vi "Zeiss File Header.vi"(0 "refnum":refnum<file>, 1 "Notes":string, 2 "Other detectors":T1, 5 "task":refnum<k21>, 7 "Resolution and scan":T5={"X resolution"=1, "Y resolution"=1, "AI oversampling"=1, "Read AI delay"=1, "Scan speed"=1, "Actual AO rate"=1.0, "Frame line rampdown ratio"=1.0, "X min (V)"=0.0, "X max (V)"=0.0}, 9 "AI channels":T4, 11 "error in":errorcluster, 12 "SEM parameters":T2={"Detector A"="", "Detector B"="Detecter B name", "Brightness A"=0.0, "Contrast A"=0.0, "Brightness B"=0.0, "Contrast B"=0.0, "Magnification"=0.0, "Pixel size"=0.0, "Working distance"=0.0, "EHT"=0.0, "Aperture"=0, "High current mode"=0, "Probe current"=0.0, "Scan rotation"=0.0, "Chamber vac"=0.0, "Gun vac"=0.0, "Beam shift X"=0.0, "Beam shift Y"=0.0, "Stig X"=0.0, "Stig Y"=0.0, "Alignment X"=0.0, "Alignment Y"=0.0, "Stage X"=0.0, "Stage Y"=0.0, "Stage Z"=0.0, "Stage T"=0.0, "Stage R"=0.0, "Stage M"=0.0}, 13 "FIB parameters":T3) -> (4 "dup refnum":refnum<file>, 6 "task out":refnum<k21>, 15 "error out":errorcluster)   [LabVIEW 2012]
uses:
  <resource>/objmgr/daqmx.rc
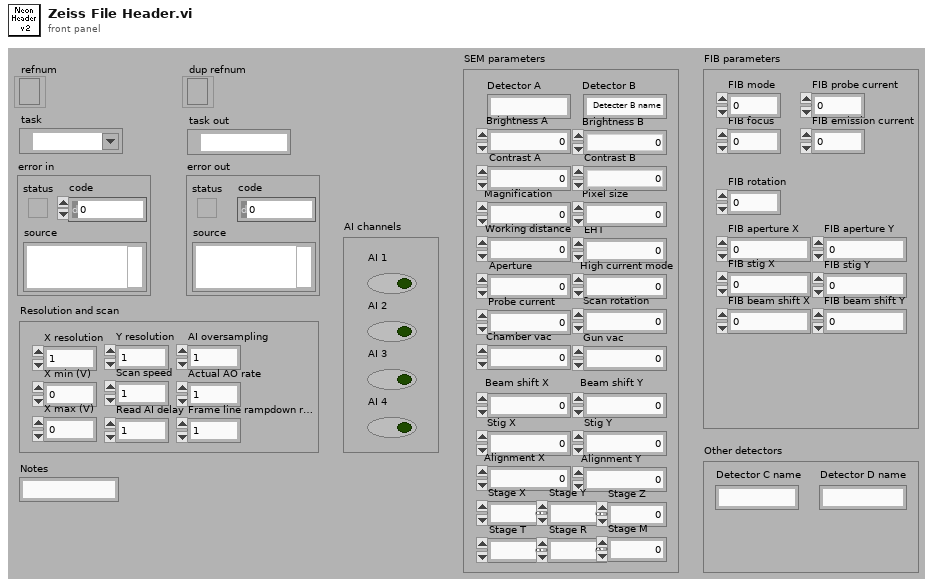
[diagram p1: front panel]
types:
  T1 = cluster{"Detector C name":string, "Detector D name":string}
  T2 = cluster{"Detector A":string, "Detector B":string, "Brightness A":sgl, "Contrast A":sgl, "Brightness B":sgl, "Contrast B":sgl, "Magnification":sgl, "Pixel size":sgl, "Working distance":sgl, "EHT":sgl, "Aperture":u8, "High current mode":u8, "Probe current":sgl, "Scan rotation":sgl, "Chamber vac":sgl, "Gun vac":sgl, "Beam shift X":sgl, "Beam shift Y":sgl, "Stig X":sgl, "Stig Y":sgl, "Alignment X":sgl, "Alignment Y":sgl, "Stage X":sgl, "Stage Y":sgl, "Stage Z":sgl, "Stage T":sgl, "Stage R":sgl, "Stage M":sgl}
  T3 = cluster{"FIB mode":u8, "FIB focus":sgl, "FIB probe current":u8, "FIB emission current":sgl, "FIB rotation":sgl, "FIB aperture X":sgl, "FIB aperture Y":sgl, "FIB stig X":sgl, "FIB stig Y":sgl, "FIB beam shift X":sgl, "FIB beam shift Y":sgl}
  T4 = cluster{"AI 1":bool, "AI 2":bool, "AI 3":bool, "AI 4":bool}
  T5 = cluster{"X resolution":u32, "Y resolution":u32, "AI oversampling":u16, "Read AI delay":i16, "Scan speed":u8, "Actual AO rate":dbl, "Frame line rampdown ratio":dbl, "X min (V)":dbl, "X max (V)":dbl}
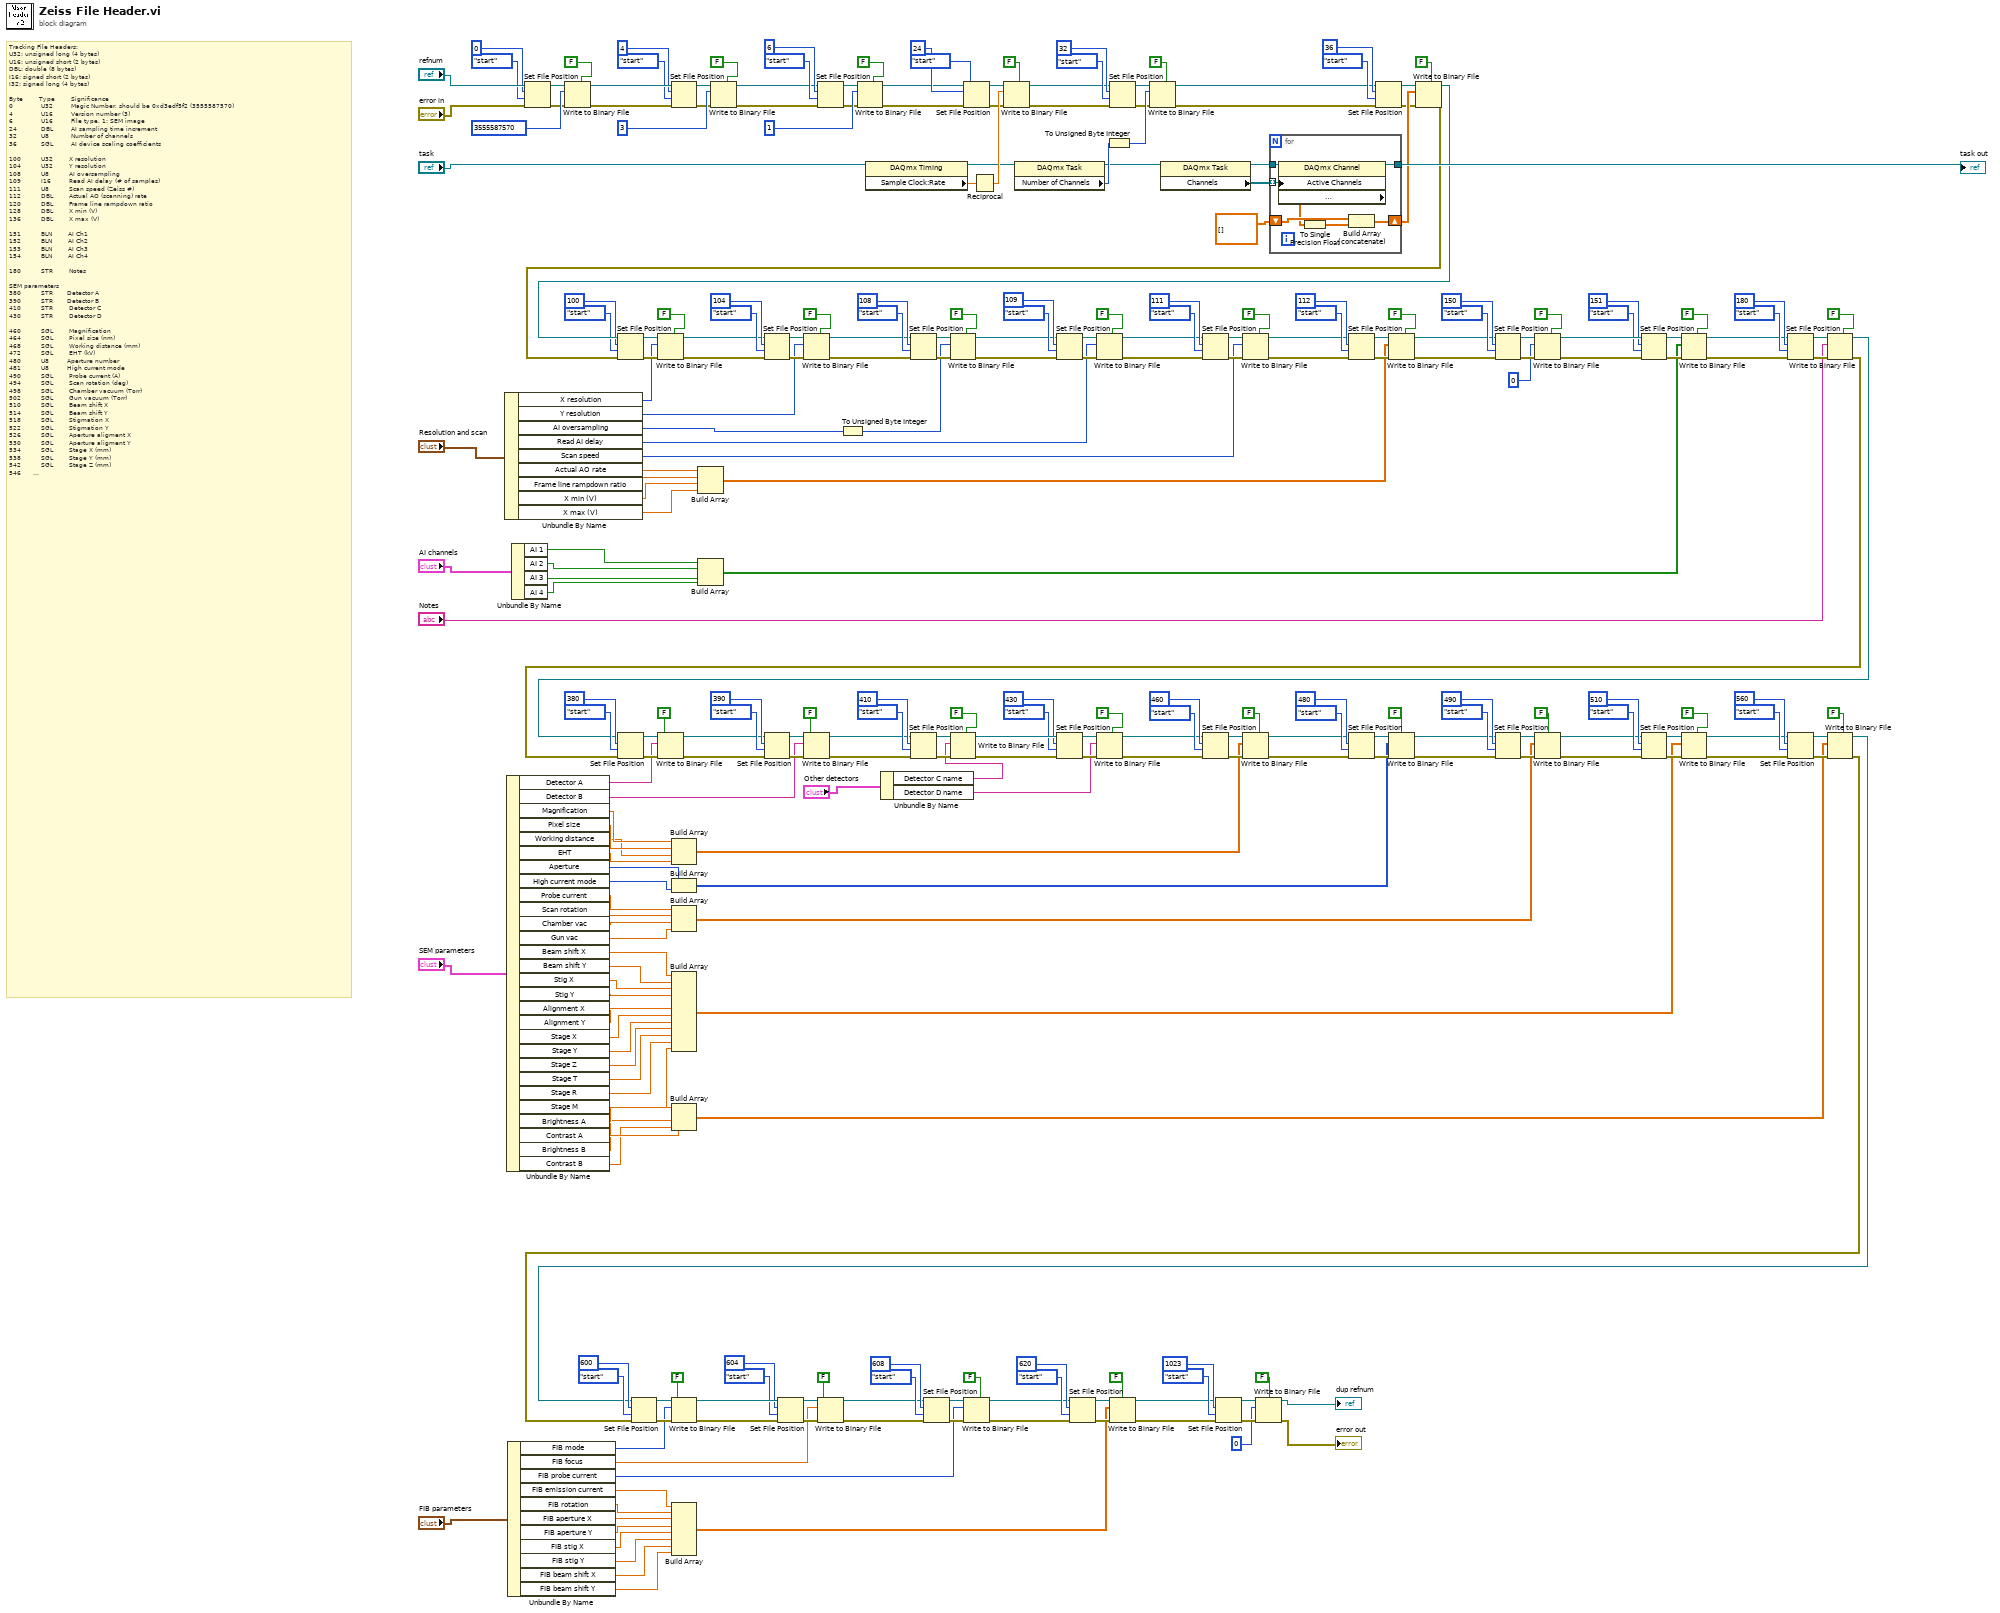
[diagram p0: block diagram]
diagram:
  # "Tracking File Headers:\nU32: unsigned long (4 bytes)\nU16: unsigned short (2 bytes)\nDBL: double (8 bytes)\nI16: signed short (2 bytes)\nI32: signed long (4 bytes)\n\nByte\t       Type\t\t      Significance\n0              U32\t        Magic Number, should be 0xd3edf5f2 (3555587570)\n4   \t          U16\t        Version number (3)\n6   \t          U16\t        File type. 1: SEM image\n24     \t      DBL         AI sampling time increment\n32     \t      U8           Number of channels\n36            SGL         AI device scaling coefficients\n\n100          U32        X resolution\n104          U32        Y resolution\n108          U8          AI oversampling\n109          I16         Read AI delay (# of samples)\n111          U8          Scan speed (Zeiss #)\n112          DBL        Actual AO (scanning) rate\n120          DBL        Frame line rampdown ratio\n128          DBL        X min (V)\n136          DBL        X max (V)\n\n151          BLN        AI Ch1          \n152          BLN        AI Ch2\n153          BLN        AI Ch3\n154          BLN        AI Ch4\n \n180          STR        Notes\n\nSEM parameters\n380          STR       Detector A\n390          STR       Detector B\n410          STR        Detector C\n430          STR        Detector D\n\n460          SGL        Magnification\n464          SGL        Pixel size (nm)\n468          SGL        Working distance (mm)\n472          SGL        EHT (kV)\n480          U8         Aperture number\n481          U8         High current mode\n490          SGL        Probe current (A)\n494          SGL        Scan rotation (deg)\n498          SGL        Chamber vacuum (Torr)\n502          SGL        Gun vacuum (Torr)\n510          SGL        Beam shift X\n514          SGL        Beam shift Y\n518          SGL        Stigmation X\n522          SGL        Stigmation Y\n526          SGL        Aperture aligment X\n530          SGL        Aperture aligment Y\n534          SGL        Stage X (mm)\n538          SGL        Stage Y (mm)\n542          SGL        Stage Z (mm)\n546          SGL        Stage T (deg)\n550          SGL        Stage R (deg)\n554          SGL        Stage M (mm)\n560          SGL        Brightness (%), detector A\n564          SGL        Contrast (%),  detector A\n568          SGL        Brightness (%), detector B\n572          SGL        Contrast (%),  detector B\n\n\nFIB parameters\n600          U8         Mode\n604          SGL        Focus (V)\n608          U8         Probe current number\n620          SGL        Emission current (A)\n624          SGL        rotation (deg)\n628          SGL        Aperture alignment X\n632          SGL        Aperture alignment Y\n636          SGL        Stigmation X\n640          SGL        Stigmation Y\n644          SGL        Beam shift X (um)\n648          SGL        Beam shift Y (um)\n\n\n1000        DBL         File length\n\n1024        I16          1-D array of n channels of unscaled measurement from DAQ"
  n1 = Unbundle By Name("Resolution and scan") -> ("X resolution"=w177:u32, "Y resolution"=w176:u32, "AI oversampling"=w175:u16, "Read AI delay"=w174:i16, "Scan speed"=w173:u8, "Actual AO rate"=w79:dbl, "Frame line rampdown ratio"=w78:dbl, "X min (V)"=w77:dbl, "X max (V)"=w76:dbl)
  n2 = Unbundle By Name("SEM parameters") -> ("Detector A"=w86:string, "Detector B"=w85:string, "Magnification"=w35:sgl, "Pixel size"=w34:sgl, "Working distance"=w33:sgl, "EHT"=w32:sgl, "Aperture"=w95:u8, "High current mode"=w94:u8, "Probe current"=w48:sgl, "Scan rotation"=w47:sgl, "Chamber vac"=w46:sgl, "Gun vac"=w45:sgl, "Beam shift X"=w71:sgl, "Beam shift Y"=w70:sgl, "Stig X"=w25:sgl, "Stig Y"=w24:sgl, "Alignment X"=w23:sgl, "Alignment Y"=w22:sgl, "Stage X"=w20:sgl, "Stage Y"=w19:sgl, "Stage Z"=w18:sgl, "Stage T"=w17:sgl, "Stage R"=w16:sgl, "Stage M"=w15:sgl, "Brightness A"=w84:sgl, "Contrast A"=w83:sgl, "Brightness B"=w81:sgl, "Contrast B"=w82:sgl)
  n3 = Unbundle By Name("FIB parameters") -> ("FIB mode"=w98:u8, "FIB focus"=w97:sgl, "FIB probe current"=w96:u8, "FIB emission current"=w12:sgl, "FIB rotation"=w11:sgl, "FIB aperture X"=w10:sgl, "FIB aperture Y"=w9:sgl, "FIB stig X"=w8:sgl, "FIB stig Y"=w7:sgl, "FIB beam shift X"=w6:sgl, "FIB beam shift Y"=w5:sgl)
  n4 = Unbundle By Name("AI channels") -> ("AI 1"=w40:bool, "AI 2"=w39:bool, "AI 3"=w38:bool, "AI 4"=w37:bool)
  n5 = Set File Position(offset (in bytes) (0)=0 ("pos offset (0)"), refnum="refnum", from (0:start)=enum16{"start", "end", "current"}."start" ("pos mode (0:2)"), error in="error in") -> (refnum out=w237:refnum<file>, error out=w236:errorcluster)
  n6 = Write to Binary File(file (use dialog)=w237, data=u32 3555587570, error in=w236, 5:FALSE ("prepend array or string size? (T)")) -> (refnum out=w289:refnum<file>, error out=w286:errorcluster)  [unwired: 3 out]
  n7 = Set File Position(offset (in bytes) (0)=4 ("pos offset (0)"), refnum=w289, from (0:start)=enum16{"start", "end", "current"}."start" ("pos mode (0:2)"), error in=w286) -> (refnum out=w240:refnum<file>, error out=w239:errorcluster)
  n8 = Build Array(w35, w34, w33, w32) -> (w31:sgl[])
  n9 = Build Array(w95, w94) -> (w28:u8[])
  n10 = Build Array(w48, w47, w46, w45) -> (w27:sgl[])
  n11 = Build Array(w71, w70, w25, w24, w23, w22, w20, w19, w18, w17, w16, w15) -> (w26:sgl[])
  n12 = Build Array(w84, w83, w81, w82) -> (w21:sgl[])
  n13 = Build Array(w12, w11, w10, w9, w8, w7, w6, w5) -> (w4:sgl[])
  n14 = Build Array(w79, w78, w77, w76) -> (w75:dbl[])
  n15 = Build Array(w40, w39, w38, w37) -> (w36:bool[])
  n16 = Write to Binary File(file (use dialog)=w240, data=u16 3, error in=w239, 5:FALSE ("prepend array or string size? (T)")) -> (refnum out=w280:refnum<file>, error out=w279:errorcluster)  [unwired: 3 out]
  n17 = Set File Position(offset (in bytes) (0)=6 ("pos offset (0)"), refnum=w280, from (0:start)=enum16{"start", "end", "current"}."start" ("pos mode (0:2)"), error in=w279) -> (refnum out=w243:refnum<file>, error out=w242:errorcluster)
  n18 = To Unsigned Byte Integer(number=w175) -> (unsigned 8bit integer=w72:u8)
  n19 = Write to Binary File(file (use dialog)=w243, data=u16 1, error in=w242, 5:FALSE ("prepend array or string size? (T)")) -> (refnum out=w275:refnum<file>, error out=w274:errorcluster)  [unwired: 3 out]
  n20 = property class="DAQmx Timing"(reference="task") -> (reference out=w271:refnum<k21>, "Sample Clock:Rate"=w273:dbl)  [unwired: 1 in, 1 out]
  n21 = Unbundle By Name("Other detectors") -> ("Detector C name"=w53:string, "Detector D name"=w52:string)
  n22 = Set File Position(offset (in bytes) (0)=24 ("pos offset (0)"), refnum=w275, from (0:start)=enum16{"start", "end", "current"}."start" ("pos mode (0:2)"), error in=w274) -> (refnum out=w246:refnum<file>, error out=w245:errorcluster)
  n23 = Reciprocal(x=w273) -> (1/x=w272:dbl)
  n24 = Write to Binary File(file (use dialog)=w246, data=w272, error in=w245, 5:FALSE ("prepend array or string size? (T)")) -> (refnum out=w268:refnum<file>, error out=w267:errorcluster)  [unwired: 3 out]
  n25 = property class="DAQmx Task"(reference=w271) -> (reference out=w265:refnum<k21>, "Number of Channels"=w266:u32)  [unwired: 1 in, 1 out]
  n26 = To Unsigned Byte Integer(number=w266) -> (unsigned 8bit integer=w258:u8)
  n27 = Set File Position(offset (in bytes) (0)=32 ("pos offset (0)"), refnum=w268, from (0:start)=enum16{"start", "end", "current"}."start" ("pos mode (0:2)"), error in=w267) -> (refnum out=w249:refnum<file>, error out=w248:errorcluster)
  n28 = Write to Binary File(file (use dialog)=w249, data=w258, error in=w248, 5:FALSE ("prepend array or string size? (T)")) -> (refnum out=w262:refnum<file>, error out=w261:errorcluster)  [unwired: 3 out]
  n29 = property class="DAQmx Task"(reference=w265) -> (reference out=w257:refnum<k21>, "Channels"=w255:refnum<k21>[])  [unwired: 1 in, 1 out]
  n30 = for {
    tunnel: [w298] -> w256
    tunnel: w257 -> [w297]
    tunnel: w255 -> [w296] mode=indexing
    shift-right: [w295] -> w254
    shift-left: sgl[][] [] -> [w294]
    n31 = property class="DAQmx Channel"(reference=w297, "Active Channels"=w296) -> (reference out=w298:refnum<k21>, "Analog Input:General Properties:Advanced:Device Scaling Coefficients:Device Scaling Coefficients"=w293:dbl[])  [unwired: 1 in, 1 out]
    n32 = To Single Precision Float(number=w293) -> (single precision float=w292:sgl[])
    n33 = Build Array (concatenate)(w294, w292) -> (w295:sgl[][])
  }
  "task out" <- w256
  n34 = Set File Position(offset (in bytes) (0)=36 ("pos offset (0)"), refnum=w262, from (0:start)=enum16{"start", "end", "current"}."start" ("pos mode (0:2)"), error in=w261) -> (refnum out=w252:refnum<file>, error out=w251:errorcluster)
  n35 = Write to Binary File(file (use dialog)=w252, data=w254, error in=w251, 5:FALSE ("prepend array or string size? (T)")) -> (refnum out=w234:refnum<file>, error out=w233:errorcluster)  [unwired: 3 out]
  n36 = Set File Position(offset (in bytes) (0)=100 ("pos offset (0)"), refnum=w234, from (0:start)=enum16{"start", "end", "current"}."start" ("pos mode (0:2)"), error in=w233) -> (refnum out=w226:refnum<file>, error out=w227:errorcluster)
  n37 = Write to Binary File(file (use dialog)=w226, data=w177, error in=w227, 5:FALSE ("prepend array or string size? (T)")) -> (refnum out=w203:refnum<file>, error out=w202:errorcluster)  [unwired: 3 out]
  n38 = Set File Position(offset (in bytes) (0)=104 ("pos offset (0)"), refnum=w203, from (0:start)=enum16{"start", "end", "current"}."start" ("pos mode (0:2)"), error in=w202) -> (refnum out=w219:refnum<file>, error out=w218:errorcluster)
  n39 = Write to Binary File(file (use dialog)=w219, data=w176, error in=w218, 5:FALSE ("prepend array or string size? (T)")) -> (refnum out=w205:refnum<file>, error out=w204:errorcluster)  [unwired: 3 out]
  n40 = Set File Position(offset (in bytes) (0)=108 ("pos offset (0)"), refnum=w205, from (0:start)=enum16{"start", "end", "current"}."start" ("pos mode (0:2)"), error in=w204) -> (refnum out=w216:refnum<file>, error out=w217:errorcluster)
  n41 = Write to Binary File(file (use dialog)=w216, data=w72, error in=w217, 5:FALSE ("prepend array or string size? (T)")) -> (refnum out=w207:refnum<file>, error out=w206:errorcluster)  [unwired: 3 out]
  n42 = Set File Position(offset (in bytes) (0)=109 ("pos offset (0)"), refnum=w207, from (0:start)=enum16{"start", "end", "current"}."start" ("pos mode (0:2)"), error in=w206) -> (refnum out=w209:refnum<file>, error out=w208:errorcluster)
  n43 = Write to Binary File(file (use dialog)=w209, data=w174, error in=w208, 5:FALSE ("prepend array or string size? (T)")) -> (refnum out=w196:refnum<file>, error out=w195:errorcluster)  [unwired: 3 out]
  n44 = Set File Position(offset (in bytes) (0)=111 ("pos offset (0)"), refnum=w196, from (0:start)=enum16{"start", "end", "current"}."start" ("pos mode (0:2)"), error in=w195) -> (refnum out=w198:refnum<file>, error out=w197:errorcluster)
  n45 = Write to Binary File(file (use dialog)=w198, data=w173, error in=w197, 5:FALSE ("prepend array or string size? (T)")) -> (refnum out=w189:refnum<file>, error out=w188:errorcluster)  [unwired: 3 out]
  n46 = Set File Position(offset (in bytes) (0)=112 ("pos offset (0)"), refnum=w189, from (0:start)=enum16{"start", "end", "current"}."start" ("pos mode (0:2)"), error in=w188) -> (refnum out=w193:refnum<file>, error out=w194:errorcluster)
  n47 = Write to Binary File(file (use dialog)=w193, data=w75, error in=w194, 5:FALSE ("prepend array or string size? (T)")) -> (refnum out=w182:refnum<file>, error out=w181:errorcluster)  [unwired: 3 out]
  n48 = Set File Position(offset (in bytes) (0)=150 ("pos offset (0)"), refnum=w182, from (0:start)=enum16{"start", "end", "current"}."start" ("pos mode (0:2)"), error in=w181) -> (refnum out=w186:refnum<file>, error out=w187:errorcluster)
  n49 = Write to Binary File(file (use dialog)=w186, data=0 ("pos offset (0)"), error in=w187, 5:FALSE ("prepend array or string size? (T)")) -> (refnum out=w180:refnum<file>, error out=w179:errorcluster)  [unwired: 3 out]
  n50 = Set File Position(offset (in bytes) (0)=151 ("pos offset (0)"), refnum=w180, from (0:start)=enum16{"start", "end", "current"}."start" ("pos mode (0:2)"), error in=w179) -> (refnum out=w164:refnum<file>, error out=w163:errorcluster)
  n51 = Write to Binary File(file (use dialog)=w164, data=w36, error in=w163, 5:FALSE ("prepend array or string size? (T)")) -> (refnum out=w42:refnum<file>, error out=w41:errorcluster)  [unwired: 3 out]
  n52 = Set File Position(offset (in bytes) (0)=180 ("pos offset (0)"), refnum=w42, from (0:start)=enum16{"start", "end", "current"}."start" ("pos mode (0:2)"), error in=w41) -> (refnum out=w169:refnum<file>, error out=w168:errorcluster)
  n53 = Write to Binary File(file (use dialog)=w169, data="Notes", error in=w168, 5:FALSE ("prepend array or string size? (T)")) -> (refnum out=w44:refnum<file>, error out=w43:errorcluster)  [unwired: 3 out]
  n54 = Set File Position(offset (in bytes) (0)=380 ("pos offset (0)"), refnum=w44, from (0:start)=enum16{"start", "end", "current"}."start" ("pos mode (0:2)"), error in=w43) -> (refnum out=w140:refnum<file>, error out=w139:errorcluster)
  n55 = Write to Binary File(file (use dialog)=w140, data=w86, error in=w139, 5:FALSE ("prepend array or string size? (T)")) -> (refnum out=w88:refnum<file>, error out=w87:errorcluster)  [unwired: 3 out]
  n56 = Set File Position(offset (in bytes) (0)=390 ("pos offset (0)"), refnum=w88, from (0:start)=enum16{"start", "end", "current"}."start" ("pos mode (0:2)"), error in=w87) -> (refnum out=w91:refnum<file>, error out=w90:errorcluster)
  n57 = Write to Binary File(file (use dialog)=w91, data=w85, error in=w90, 5:FALSE ("prepend array or string size? (T)")) -> (refnum out=w57:refnum<file>, error out=w56:errorcluster)  [unwired: 3 out]
  n58 = Set File Position(offset (in bytes) (0)=410 ("pos offset (0)"), refnum=w57, from (0:start)=enum16{"start", "end", "current"}."start" ("pos mode (0:2)"), error in=w56) -> (refnum out=w66:refnum<file>, error out=w67:errorcluster)
  n59 = Write to Binary File(file (use dialog)=w66, data=w53, error in=w67, 5:FALSE ("prepend array or string size? (T)")) -> (refnum out=w68:refnum<file>, error out=w69:errorcluster)  [unwired: 3 out]
  n60 = Set File Position(offset (in bytes) (0)=430 ("pos offset (0)"), refnum=w68, from (0:start)=enum16{"start", "end", "current"}."start" ("pos mode (0:2)"), error in=w69) -> (refnum out=w59:refnum<file>, error out=w58:errorcluster)
  n61 = Write to Binary File(file (use dialog)=w59, data=w52, error in=w58, 5:FALSE ("prepend array or string size? (T)")) -> (refnum out=w55:refnum<file>, error out=w54:errorcluster)  [unwired: 3 out]
  n62 = Set File Position(offset (in bytes) (0)=460 ("pos offset (0)"), refnum=w55, from (0:start)=enum16{"start", "end", "current"}."start" ("pos mode (0:2)"), error in=w54) -> (refnum out=w143:refnum<file>, error out=w142:errorcluster)
  n63 = Write to Binary File(file (use dialog)=w143, data=w31, error in=w142, 5:FALSE ("prepend array or string size? (T)")) -> (refnum out=w155:refnum<file>, error out=w154:errorcluster)  [unwired: 3 out]
  n64 = Set File Position(offset (in bytes) (0)=480 ("pos offset (0)"), refnum=w155, from (0:start)=enum16{"start", "end", "current"}."start" ("pos mode (0:2)"), error in=w154) -> (refnum out=w146:refnum<file>, error out=w145:errorcluster)
  n65 = Write to Binary File(file (use dialog)=w146, data=w28, error in=w145, 5:FALSE ("prepend array or string size? (T)")) -> (refnum out=w151:refnum<file>, error out=w150:errorcluster)  [unwired: 3 out]
  n66 = Set File Position(offset (in bytes) (0)=490 ("pos offset (0)"), refnum=w151, from (0:start)=enum16{"start", "end", "current"}."start" ("pos mode (0:2)"), error in=w150) -> (refnum out=w149:refnum<file>, error out=w148:errorcluster)
  n67 = Write to Binary File(file (use dialog)=w149, data=w27, error in=w148, 5:FALSE ("prepend array or string size? (T)")) -> (refnum out=w30:refnum<file>, error out=w29:errorcluster)  [unwired: 3 out]
  n68 = Set File Position(offset (in bytes) (0)=510 ("pos offset (0)"), refnum=w30, from (0:start)=enum16{"start", "end", "current"}."start" ("pos mode (0:2)"), error in=w29) -> (refnum out=w136:refnum<file>, error out=w137:errorcluster)
  n69 = Write to Binary File(file (use dialog)=w136, data=w26, error in=w137, 5:FALSE ("prepend array or string size? (T)")) -> (refnum out=w50:refnum<file>, error out=w49:errorcluster)  [unwired: 3 out]
  n70 = Set File Position(offset (in bytes) (0)=560 ("pos offset (0)"), refnum=w50, from (0:start)=enum16{"start", "end", "current"}."start" ("pos mode (0:2)"), error in=w49) -> (refnum out=w230:refnum<file>, error out=w231:errorcluster)
  n71 = Write to Binary File(file (use dialog)=w230, data=w21, error in=w231, 5:FALSE ("prepend array or string size? (T)")) -> (refnum out=w13:refnum<file>, error out=w14:errorcluster)  [unwired: 3 out]
  n72 = Set File Position(offset (in bytes) (0)=600 ("pos offset (0)"), refnum=w13, from (0:start)=enum16{"start", "end", "current"}."start" ("pos mode (0:2)"), error in=w14) -> (refnum out=w130:refnum<file>, error out=w131:errorcluster)
  n73 = Write to Binary File(file (use dialog)=w130, data=w98, error in=w131, 5:FALSE ("prepend array or string size? (T)")) -> (refnum out=w127:refnum<file>, error out=w126:errorcluster)  [unwired: 3 out]
  n74 = Set File Position(offset (in bytes) (0)=604 ("pos offset (0)"), refnum=w127, from (0:start)=enum16{"start", "end", "current"}."start" ("pos mode (0:2)"), error in=w126) -> (refnum out=w102:refnum<file>, error out=w101:errorcluster)
  n75 = Write to Binary File(file (use dialog)=w102, data=w97, error in=w101, 5:FALSE ("prepend array or string size? (T)")) -> (refnum out=w121:refnum<file>, error out=w120:errorcluster)  [unwired: 3 out]
  n76 = Set File Position(offset (in bytes) (0)=608 ("pos offset (0)"), refnum=w121, from (0:start)=enum16{"start", "end", "current"}."start" ("pos mode (0:2)"), error in=w120) -> (refnum out=w105:refnum<file>, error out=w104:errorcluster)
  n77 = Write to Binary File(file (use dialog)=w105, data=w96, error in=w104, 5:FALSE ("prepend array or string size? (T)")) -> (refnum out=w117:refnum<file>, error out=w116:errorcluster)  [unwired: 3 out]
  n78 = Set File Position(offset (in bytes) (0)=620 ("pos offset (0)"), refnum=w117, from (0:start)=enum16{"start", "end", "current"}."start" ("pos mode (0:2)"), error in=w116) -> (refnum out=w108:refnum<file>, error out=w107:errorcluster)
  n79 = Write to Binary File(file (use dialog)=w108, data=w4, error in=w107, 5:FALSE ("prepend array or string size? (T)")) -> (refnum out=w113:refnum<file>, error out=w112:errorcluster)  [unwired: 3 out]
  n80 = Set File Position(offset (in bytes) (0)=1023 ("pos offset (0)"), refnum=w113, from (0:start)=enum16{"start", "end", "current"}."start" ("pos mode (0:2)"), error in=w112) -> (refnum out=w111:refnum<file>, error out=w110:errorcluster)
  n81 = Write to Binary File(file (use dialog)=w111, data=i8 0, error in=w110, 5:FALSE ("prepend array or string size? (T)")) -> (refnum out=→"dup refnum":refnum<file>, error out=→"error out":errorcluster)  [unwired: 3 out]
